vi "inicjalizacja.vi"() -> (0 "Error":errorcluster, 3 "Lista komór":T1[](array[typedef]))   [LabVIEW 2014]
uses:
  glownaMaszynaStanowVIs/wykonajRuchVIs/parametryKomorVIs/WyborKomory.ctl
  glownaMaszynaStanowVIs/AkcjaGFV.ctl
  <vilib>/MakerHub/LINX/Public/Utilities/Open Local.vi
  <vilib>/MakerHub/LINX/LMH-LINX.lvlib
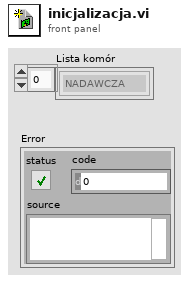
[diagram p1: front panel]
types:
  T1 = typedef "WyborKomory.ctl" = enum16{"NADAWCZA", "ODBIORCZA"}
  T2 = typedef "AkcjaGFV.ctl" = enum16{"Czytaj", "Zapisz", "Reset"}
  T3 = typedef "LMH-LINX.lvlib/LINX Ref.ctl" = cluster{"IO":T4, "Interface":T5, "LINX Device Config":T6}
  T4 = typedef "LMH-LINX.lvlib/Platform.ctl" = enum16{"Remote", "Local"}
  T5 = typedef "LMH-LINX.lvlib/Interface.ctl" = enum16{"Serial", "TCP"}
  T6 = typedef "LMH-LINX.lvlib/Device.lvlib/LINX Device Config.ctl" = cluster{"Interface":T5, "COM Port":refnum<visa-resource-name>, "TCP Configuration":T7, "Device Family":u8, "Device ID":u8, "Device Name":string, "TCP Ref":refnum<k5>, "Channels":T8}
  T7 = typedef "LMH-LINX.lvlib/Device.lvlib/TCP Config.ctl" = cluster{"IP Address":string, "Port":u16}
  T8 = typedef "LMH-LINX.lvlib/Channels.ctl" = cluster{"DI":u8[], "DO":u8[], "AI":u8[], "AO":u8[], "PWM":u8[], "QE":u8[], "UART":u8[], "I2C 2":u8[], "SPI":u8[], "CAN":u8[], "Servo":u8[], "AI Ref (V)":dbl, "AI Resolution (Bits)":u8, "AO Ref (V)":dbl, "AO Resolution (Bits)":u8}
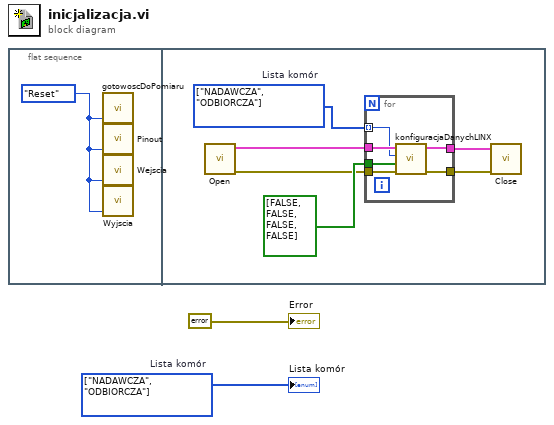
[diagram p0: block diagram]
diagram:
  w2 = T1[] [enum."NADAWCZA", enum."ODBIORCZA"] items=["NADAWCZA", "ODBIORCZA"]  # Lista komór
  n1 = flat-sequence {
    frame #0 {
      w3 = AkcjaGFV."Reset" ("Akcja")
      n2 = call "gotowoscDoPomiaru.vi"("Akcja"=w3) -> ()  [unwired: 4 in, 1 out]
      n3 = call "Pinout.vi"("Akcja"=w3) -> ()  [unwired: 4 in, 1 out]
      n4 = call "Wejscia.vi"("Akcja"=w3) -> ()  [unwired: 4 in, 1 out]
      n5 = call "Wyjscia.vi"("Akcja"=w3) -> ()  [unwired: 4 in, 1 out]
    }
    frame #1 {
      w7 = T1[] [enum."NADAWCZA", enum."ODBIORCZA"] items=["NADAWCZA", "ODBIORCZA"]  # Lista komór
      n6 = call-poly <vilib>:"Open.vi"() -> ("Error Out"=w5:errorcluster, "LINX Resource"=w4:T3)  [unwired: 9 in, 1 out]
      n7 = for {
        tunnel: w4 -> [w15]
        tunnel: w5 -> [w14]
        tunnel: bool[] [FALSE, FALSE, FALSE, FALSE] ("Kierunki") -> [w13]
        tunnel: w7 -> [w12] mode=indexing
        tunnel: [w11] -> w8
        tunnel: [w10] -> w9
        n8 = call "konfiguracjaDanychLINX.vi"("Error In"=w14, "Kierunki"=w13, "Wybór komory"=w12, "LINX Resource"=w15) -> ("Error Out"=w10:errorcluster, "LINX Out"=w11:T3)  [unwired: 6 in]
      }
      n9 = call <vilib>:"Close.vi"("Error In"=w9, "LINX Resource"=w8) -> ()  [unwired: 9 in, 1 out]
    }
  }
  "Lista komór" <- w2
  "Error" <- errorcluster {"status"=FALSE, "code"=0, "source"=""} ("Error")
